vi "zad2.vi"() -> ()   [LabVIEW 2017]
panel:
  in  "stop":bool
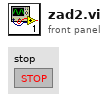
[diagram p1: front panel]
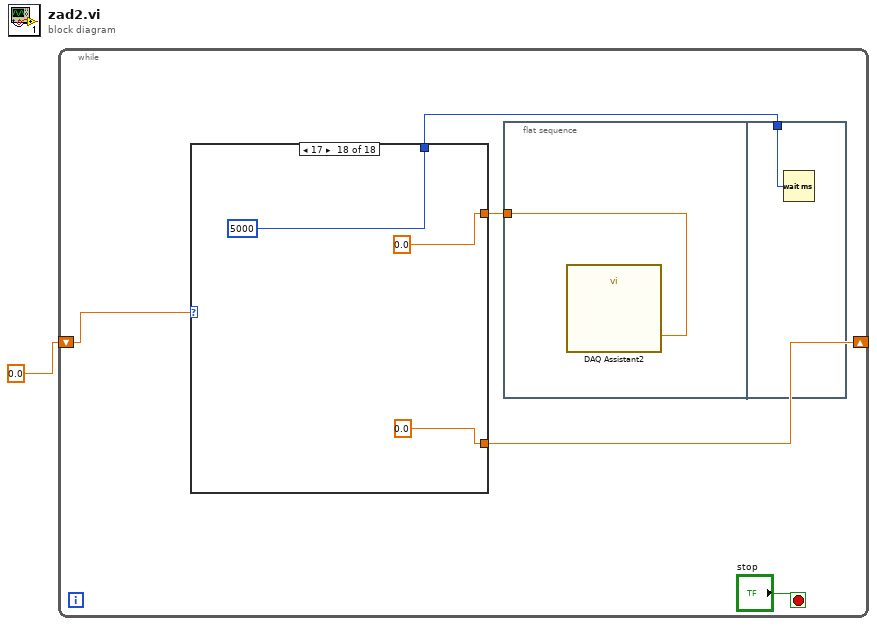
[diagram p0: block diagram]
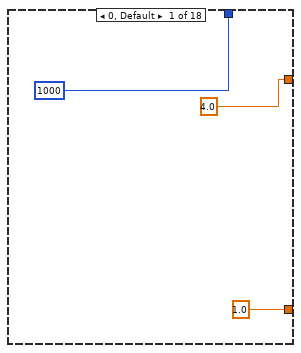
[diagram p2: hidden frame]
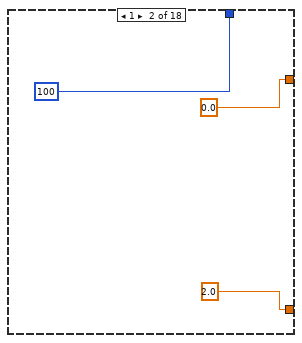
[diagram p3: hidden frame]
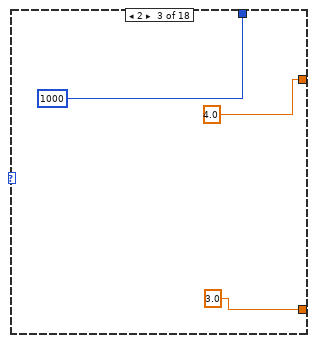
[diagram p4: hidden frame]
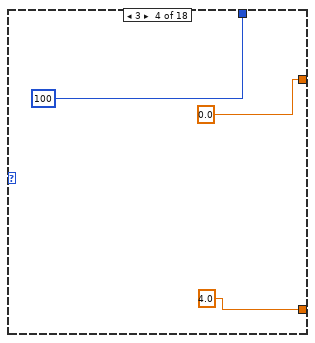
[diagram p5: hidden frame]
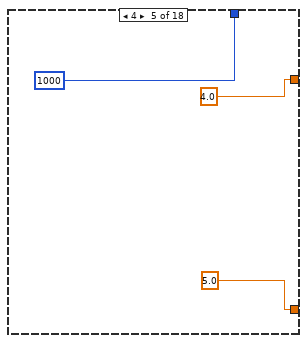
[diagram p6: hidden frame]
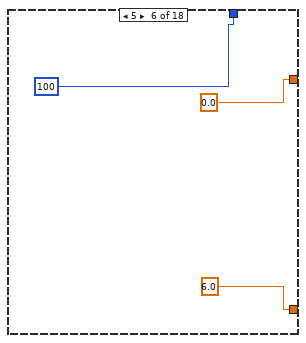
[diagram p7: hidden frame]
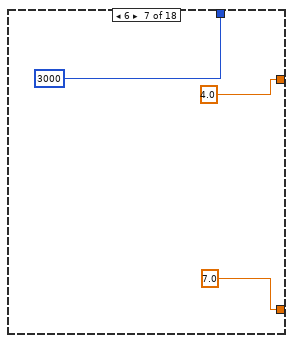
[diagram p8: hidden frame]
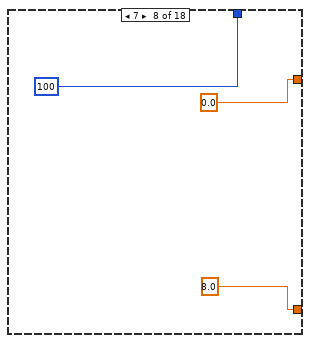
[diagram p9: hidden frame]
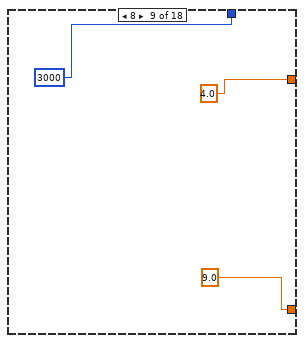
[diagram p10: hidden frame]
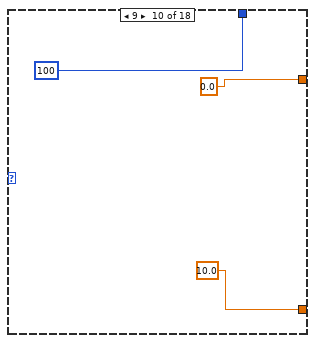
[diagram p11: hidden frame]
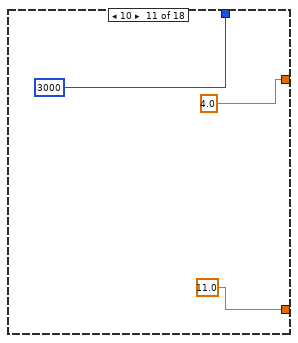
[diagram p12: hidden frame]
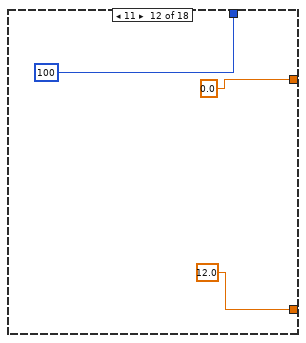
[diagram p13: hidden frame]
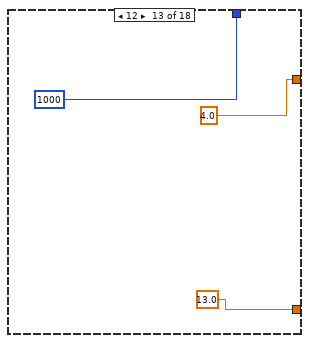
[diagram p14: hidden frame]
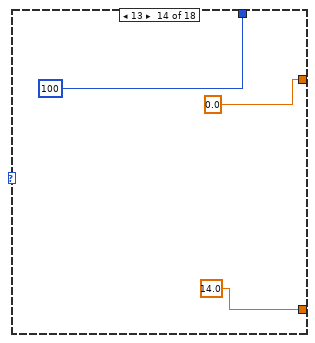
[diagram p15: hidden frame]
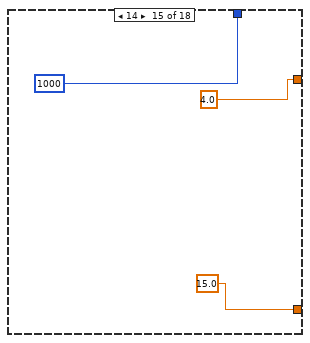
[diagram p16: hidden frame]
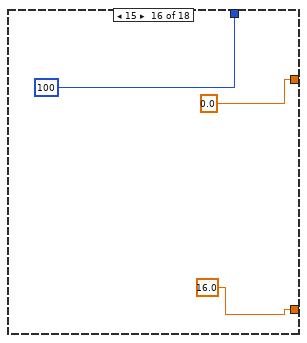
[diagram p17: hidden frame]
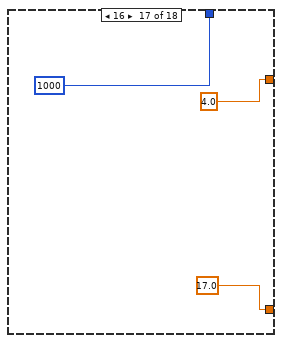
[diagram p18: hidden frame]
diagram:
  n1 = while {
    shift-right: [w4] -> _
    shift-left: 0.0 ("data") -> [w3]
    stop <- "stop" stop-if-true
    n2 = case shown="17" w3 {
      tunnel: [4.0 ("data") 0.0 ("data") 4.0 ("data") 0.0 ("data") 4.0 ("data") 0.0 ("data") 4.0 ("data") 0.0 ("data") 4.0 ("data") 0.0 ("data") 4.0 ("data") 0.0 ("data") 4.0 ("data") 0.0 ("data") 4.0 ("data") 0.0 ("data") 4.0 ("data") 0.0 ("data")] -> w5
      tunnel: [1.0 ("data") 2.0 ("data") 3.0 ("data") 4.0 ("data") 5.0 ("data") 6.0 ("data") 7.0 ("data") 8.0 ("data") 9.0 ("data") 10.0 ("data") 11.0 ("data") 12.0 ("data") 13.0 ("data") 14.0 ("data") 15.0 ("data") 16.0 ("data") 17.0 ("data") 0.0 ("data")] -> w4
      tunnel: [1000 100 1000 100 1000 100 3000 100 3000 100 3000 100 1000 100 1000 100 1000 5000] -> w2
      frame 0, Default {
      }
      frame 1 {
      }
      frame 2 {
      }
      frame 3 {
      }
      frame 4 {
      }
      frame 5 {
      }
      frame 6 {
      }
      frame 7 {
      }
      frame 8 {
      }
      frame 9 {
      }
      frame 10 {
      }
      frame 11 {
      }
      frame 12 {
      }
      frame 13 {
      }
      frame 14 {
      }
      frame 15 {
      }
      frame 16 {
      }
      frame 17 {
      }
    }
    n3 = flat-sequence {
      tunnel: w5 -> [w7]
      tunnel: w2 -> [w8]
      frame #0 {
        n4 = call "DAQ Assistant2"("data"=w7) -> ()  [unwired: 17 in, 2 out]
      }
      frame #1 {
        n5 = Wait (ms)(milliseconds to wait=w8) -> ()  [unwired: 1 out]
      }
    }
  }
